vi "sReadArduinoParams.vi"(8 "error in":errorcluster, 11 "VISA Refnum in":refnum<visa-resource-name>) -> (0 "error out":errorcluster, 1 "Bytes read":u32, 2 "read buffer":string, 3 "VISA Refnum out":refnum<visa-resource-name>)   [LabVIEW 2014]
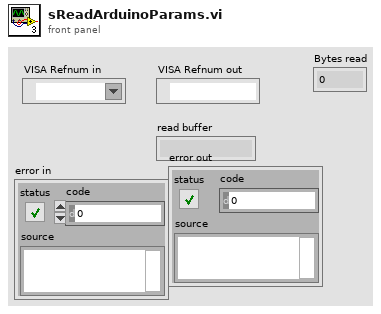
[diagram p1: front panel]
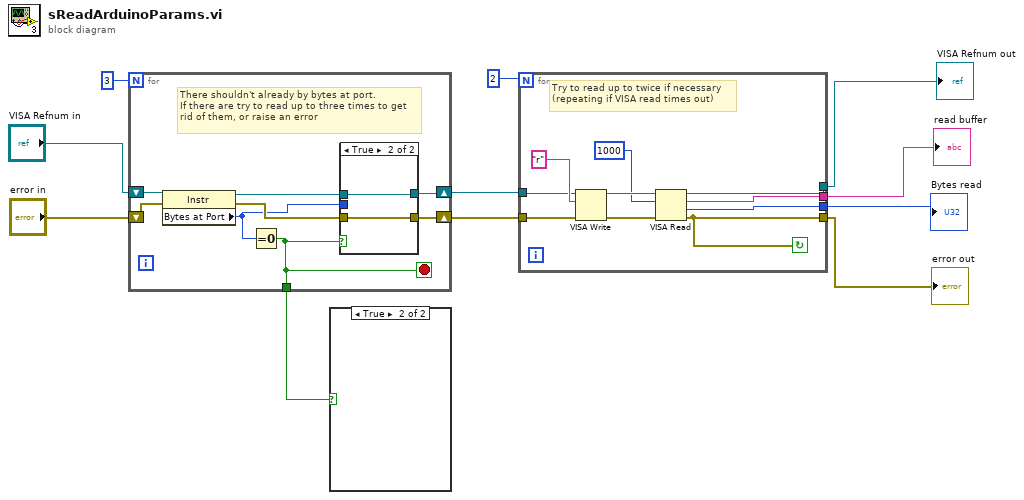
[diagram p0: block diagram]
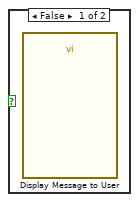
[diagram p2: hidden frame]
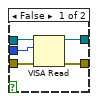
[diagram p3: hidden frame]
diagram:
  n1 = for {
    N: 3 -> [_]
    shift-right: [w14] -> w6
    shift-left: "VISA Refnum in" -> [w19]
    shift-right: [w15] -> w4
    shift-left: "error in" -> [w18]
    tunnel: [w13] -> w1
    stop <- w13 stop-if-true
    # "There shouldn't already by bytes at port.\nIf there are try to read up to three times to get\nrid of them, or raise an error"
    n2 = property class="Instr"(reference=w19, error in=w18) -> (reference out=w17:refnum<visa-resource-name>, error out=w16:errorcluster, "Bytes at Port"=w12:u32)
    n3 = Equal To 0?(x=w12) -> (x = 0?=w13:bool)
    n4 = case shown="True" w13 {
      tunnel: w17 -> [w23 w25]
      tunnel: w16 -> [w22 w26]
      tunnel: [w21 w26] -> w15
      tunnel: [w24 w25] -> w14
      tunnel: w12 -> [w20 _]
      frame False {
        n5 = VISA Read(VISA resource name=w23, byte count=w20, error in (no error)=w22) -> (VISA resource name out=w24:refnum<visa-resource-name>, error out=w21:errorcluster)  [unwired: 2 out]
      }
      frame True {
      }
    }
  }
  n6 = case shown="True" w1 {
    frame False {
      n7 = call "Display Message to User"() -> ()  [unwired: 10 in, 2 out]
    }
    frame True {
    }
  }
  n8 = for {
    N: 2 -> [_]
    tunnel: [w34] -> w11
    tunnel: [w30] -> w8
    tunnel: w6 -> [w29]
    tunnel: [w32] -> w10
    tunnel: w4 -> [w28]
    tunnel: [w27] -> w9
    stop <- w27 continue-if-true
    # "Try to read up to twice if necessary\n(repeating if VISA read times out)"
    n9 = VISA Write(VISA resource name=w29, write buffer="r", error in (no error)=w28) -> (VISA resource name out=w35:refnum<visa-resource-name>, error out=w31:errorcluster)  [unwired: 1 out]
    n10 = VISA Read(VISA resource name=w35, byte count=u32 1000, error in (no error)=w31) -> (VISA resource name out=w32:refnum<visa-resource-name>, read buffer=w34:string, return count=w30:u32, error out=w27:errorcluster)
  }
  "read buffer" <- w11
  "VISA Refnum out" <- w10
  "error out" <- w9
  "Bytes read" <- w8
